vi "Open Vi.vi"(8 "error in (no error)":errorcluster caption="错误输入（无错误）", 10 "Vi Path":path) -> (0 "error out":errorcluster caption="错误输出", 1 "Exec.State":T1(ring), 2 "IsCloneVI":bool, 3 "VI*":refnum<vi>)   [LabVIEW 2016, in "PanelDataNode.lvclass"]
uses:
  PanelDataNode.lvclass
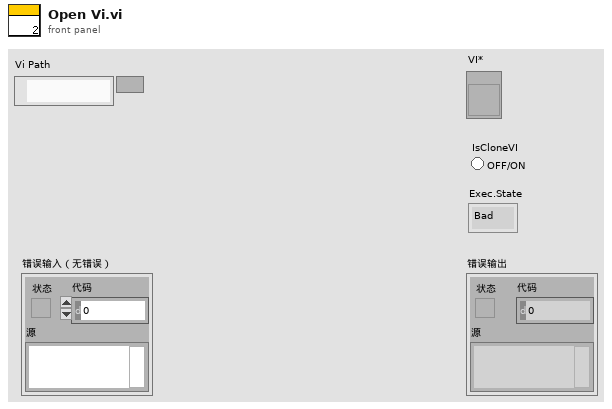
[diagram p1: front panel]
types:
  T1 = enum32{"Bad", "Idle", "Run top level", "Running"}
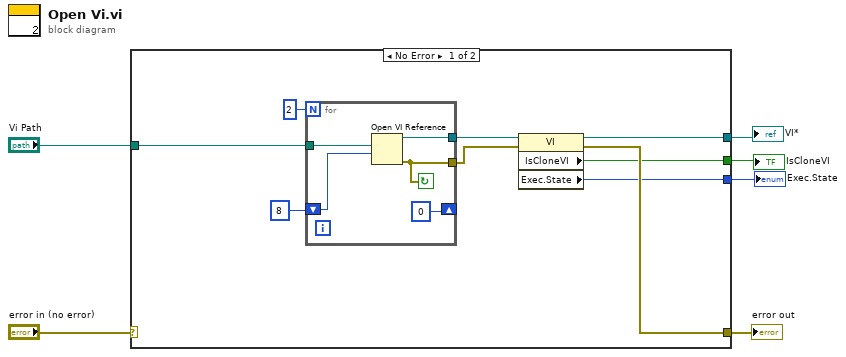
[diagram p0: block diagram]
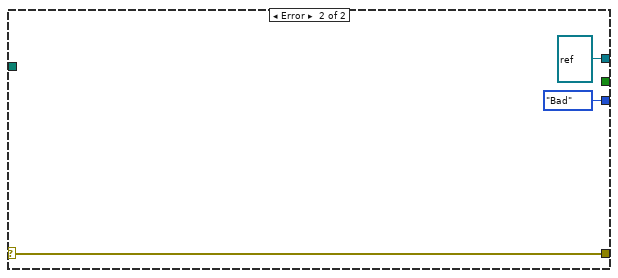
[diagram p2: hidden frame]
diagram:
  n1 = case shown="No Error" "error in (no error)" {
    selector: "error in (no error)" -> [_ w23]
    tunnel: [w9 w23] -> w5
    tunnel: "Vi Path" -> [w15 _]
    tunnel: [w11 refnum<vi> refnum ("vi reference")] -> w3
    tunnel: [w8 _] -> w2
    tunnel: [w7 T1."Bad" ("Exec.State")] -> w1
    frame No Error {
      n2 = for {
        N: 2 -> [_]
        tunnel: w15 -> [w20]
        shift-right: [0 ("选项")] -> _
        shift-left: 8 ("选项") -> [w19]
        tunnel: [w17] -> w10
        tunnel: [w16] -> w12
        stop <- w17 continue-if-true
        n3 = Open VI Reference(vi path=w20, options=w19) -> (vi reference=w16:refnum<vi>, error out=w17:errorcluster)  [unwired: 4 in]
      }
      n4 = property class="VI"(reference=w12, error in=w10) -> (reference out=w11:refnum<vi>, error out=w9:errorcluster, "IsCloneVI"=w8:bool, "Exec.State"=w7:T1)
    }
    frame Error {
    }
  }
  "error out" <- w5
  "VI*" <- w3
  "IsCloneVI" <- w2
  "Exec.State" <- w1
